vi "Load Language Files.vi"(11 "Data In":T1 {"Language" items=["English", "Español", "Português"]}) -> (3 "Data Out":T1 {"Language" items=["English", "Español", "Português"]})   [LabVIEW 2015]
uses:
  Controls/HID Data.ctl
  <vilib>/userdefined/High Color/IMAQdx.ctl
  <vilib>/vision/Image Controls.llb/IMAQ Image.ctl
  Controls/HID State.ctl
  <vilib>/Utility/file.llb/Read Delimited Spreadsheet (string).vi
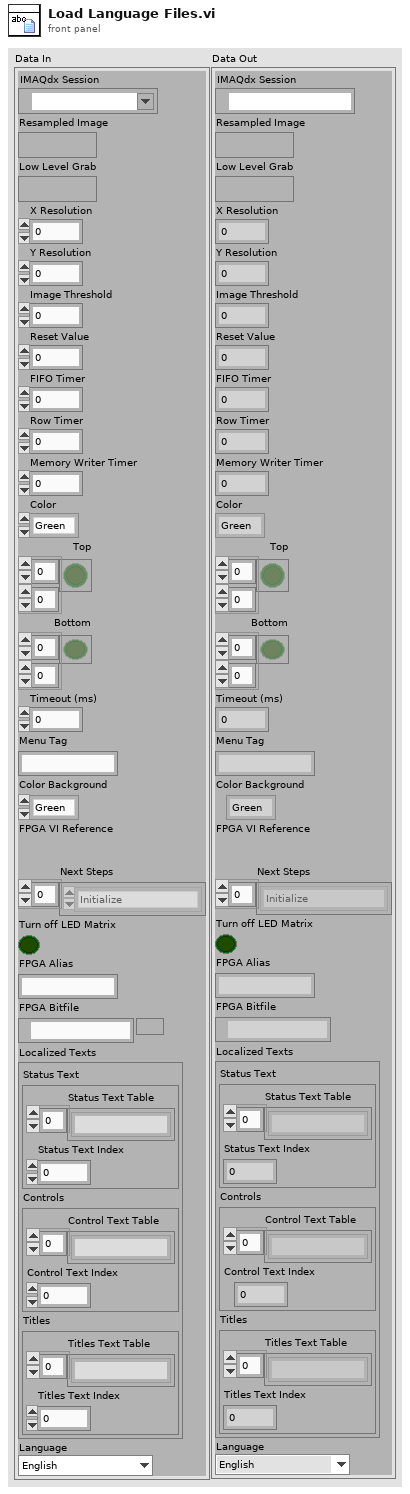
[diagram p1: front panel]
types:
  T1 = typedef "HID Data.ctl" = cluster{"IMAQdx Session":T2, "Resampled Image":T3, "Low Level Grab":T3, "X Resolution":i32, "Y Resolution":i32, "Image Threshold":u8, "Reset Value":i32, "FIFO Timer":u16, "Row Timer":u32, "Memory Writer Timer":u8, "Color":enum16{"Green", "Blue", "Red", "White", "Pink", "Yellow", "Turquoise", "Black"}, "Top":bool[][], "Bottom":bool[][], "Timeout (ms)":i32, "Menu Tag":string, "Color Background":enum16{"Green", "Blue", "Red", "White", "Pink", "Yellow", "Turquoise", "Black"}, "FPGA VI Reference":refnum<k20>, "Next Steps":T4[], "Turn off LED Matrix":bool, "FPGA Alias":string, "FPGA Bitfile":path, "Localized Texts":cluster{"Status Text":cluster{"Status Text Table":string[], "Status Text Index":i32}, "Controls":cluster{"Control Text Table":string[], "Control Text Index":i32}, "Titles":cluster{"Titles Text Table":string[], "Titles Text Index":i32}}, "Language":u16}
  T2 = typedef "IMAQdx.ctl" = refnum<k21>
  T3 = typedef "IMAQ Image.ctl" = refnum<image>
  T4 = typedef "HID State.ctl" = enum16{"Initialize", "Set FPGA Parametes", "Set Camera Parameters", "Set LED Matrix Parameters", "Initialize FPGA Interface", "Initialize Camera", "Start FPGA VI", "Start Camera", "Wait for Event", "Update UI", "Acquire", "Process Image", "Get Boolean Arrays", "Send to FPGA", "Menu Pop-Up", "Menu Actions", "Handle Errors", "Close Camera", "Close FPGA", "Stop", "Exit"}
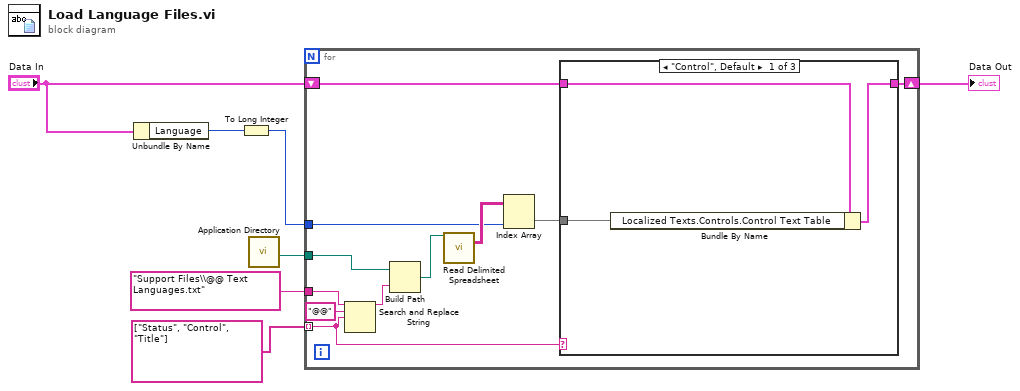
[diagram p0: block diagram]
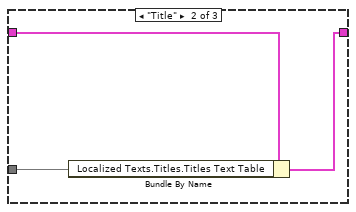
[diagram p2: hidden frame]
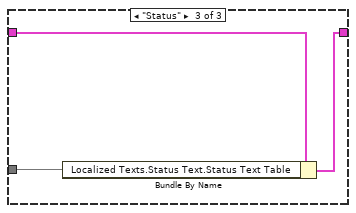
[diagram p3: hidden frame]
diagram:
  n1 = Unbundle By Name("Data In") -> ("Language"=w4:u16)
  n2 = To Long Integer(number=w4) -> (32bit integer=w5:i32)
  n3 = call <vilib>:"Application Directory.vi"() -> ("Application Directory"=w3:path)
  n4 = for {
    tunnel: w3 -> [w16]
    tunnel: w5 -> [w15]
    tunnel: "Support Files\\@@ Text Languages.txt" ("name or relative path") -> [w12]
    tunnel: string[] ["Status", "Control", "Title"] -> [w11] mode=indexing
    shift-right: [w8] -> w1
    shift-left: "Data In" -> [w9]
    n5 = Search and Replace String(input string=w12, search string="@@", replace string=w11) -> (result string=w14:string)  [unwired: 5 in, 3 out]
    n6 = Build Path(base path=w16, name or relative path=w14) -> (appended path=w17:path)
    n7 = call-poly <vilib>:"Read Delimited Spreadsheet.vi"("file path (dialog if empty)"=w17) -> ("all rows"=w18:string[][])  [unwired: 9 in, 5 out]
    n8 = Index Array(array=w18, index (col)=w15) -> (element=w10:string[])  [unwired: 1 in]
    n9 = case shown="\"Control\", Default" w11 {
      tunnel: w10 -> [w21 w24 w27]
      tunnel: w9 -> [w20 w23 w26]
      tunnel: [w19 w22 w25] -> w8
      frame "Control", Default {
        n10 = Bundle By Name(cluster=w20, "Localized Texts.Controls.Control Text Table"=w21) -> (w19:T1)
      }
      frame "Title" {
        n11 = Bundle By Name(cluster=w23, "Localized Texts.Titles.Titles Text Table"=w24) -> (w22:T1)
      }
      frame "Status" {
        n12 = Bundle By Name(cluster=w26, "Localized Texts.Status Text.Status Text Table"=w27) -> (w25:T1)
      }
    }
  }
  "Data Out" <- w1
